vi "Main Page.vi"(8 "error in (no error)":errorcluster, 11 "Node Ptr":T11 format="%.0x") -> (0 "error out":errorcluster)   [LabVIEW 2018, in "Chassis TimeSync System Explorer.lvlib"]
uses:
  Chassis TimeSync System Explorer.lvlib
  <vilib>/NI Veristand/Custom Device API/Custom Device Item Ref.ctl
  Connection Selection.ctl
  Shared/Routes.ctl
  Shared/Route.ctl
  Pins Tab.ctl
  Shared/Mode.ctl
  Shared/External Pin.ctl
  Shared/Time Reference.ctl
  Time Ref Tab.ctl
  Shared/IRIG Type.ctl
  <vilib>/NI Veristand/Custom Device API/Custom Device Channel Type.ctl
  Shared/Constants.vi
  <vilib>/NI Veristand/Custom Device API/Get Item Property (Boolean).vi
  sub_EnableDisable Control.vi
  <vilib>/NI Veristand/Custom Device API/Get Item Property (String).vi
  <vilib>/NI Veristand/Custom Device API/Get Item Property (U16).vi
  <vilib>/NI Veristand/Custom Device API/Get Item Property (Double).vi
  <vilib>/NI Veristand/Custom Device API/Set Item Property (String).vi
  <vilib>/NI Veristand/Custom Device API/Set Item Property (Boolean).vi
  <vilib>/NI Veristand/Custom Device API/Set Item Property (Variant).vi
  <vilib>/NI Veristand/Custom Device API/Set Item Property (U16).vi
  <vilib>/NI Veristand/Custom Device API/Set Item Property (I32).vi
  <vilib>/NI Veristand/Custom Device API/Set Item Property (Double).vi
  <vilib>/NI Veristand/Custom Device API/Custom Device API.lvlib
  Shared/Chassis TimeSync Shared.lvlib
panel:
  in  "6683H Warning":string
  in  "SyncModule":string caption="Chassis Clock Generation Module"
  in  "SyncModule?":bool
  in  "Settings":T1(tab)
  out "Mode Desciption":string
  in  "Mode":T2
  in  "ConSelection":T3 caption="Selection"
  out "Pins tab":T4
  in  "PFI2":bool
  in  "PFI1":bool
  in  "PFI0":bool
  in  "PXI_Trig0":bool
  in  "Route In Pin":T5
  in  "Custom Routes":T6
  out "TimeRefTab":T8
  in  "Priority 2":i32 min=0 max=255
  in  "Priority 1":i32 min=0 max=255
  in  "IRIG type":T9=enum."IRIGB AM"
  in  "Start Time":timestamp
  in  "PPSSetTime":bool
  in  "Terminal":string
  in  "Time Reference":T10
  out "Mode Desciption 2":string="When using a time reference other than PXI Backplane Clock, it is recommended to additionally configure that time refernece in Measurment and Automation Explorer (MAX) before deployment. Doing so will prevent \"macro\" adjustments to system time while the NI VeriStand engine is running."
  in  "StartDelay":u16 caption="Generation Start Delay (s)"
  in  "PhaseOffset":dbl caption="Generation Phase Offset (°)" min=0.0 max=360.0
  in  "timekeeper":string caption="Time-Based Synchronization Module"
  in  "Header":cluster{"Section Name":string}={"Section Name"="Chassis TimeSync Settings"}
  in  "Description":string
  in  "Name":string
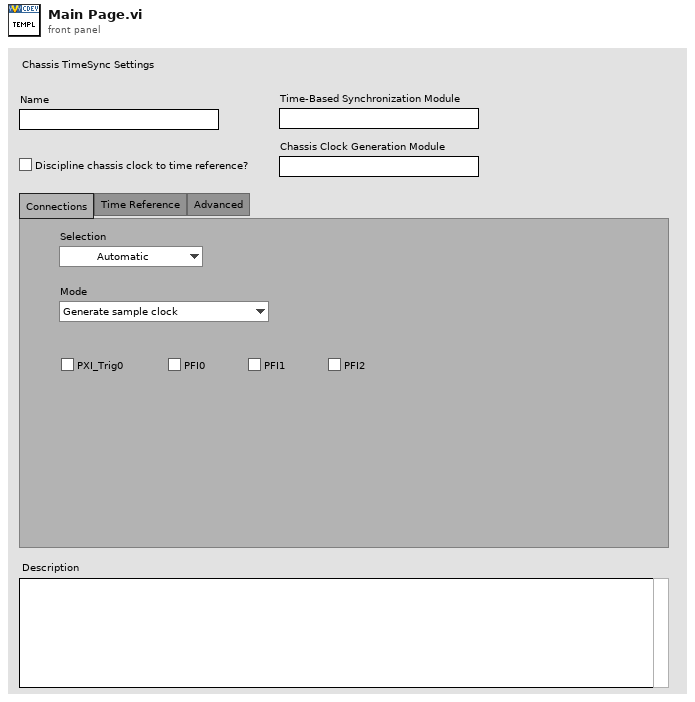
[diagram p1: front panel]
types:
  T1 = enum32{"Connections", "Time Reference", "Advanced"}
  T2 = typedef "Chassis TimeSync Shared.lvlib/Mode.ctl" = enum16{"Generate sample clock", "Route sample clock out of chassis", "Route sample clock into chassis", "Custom routes"}
  T3 = typedef "Chassis TimeSync System Explorer.lvlib/Connection Selection.ctl" = enum16{"Automatic", "Custom"}
  T4 = typedef "Chassis TimeSync System Explorer.lvlib/Pins Tab.ctl" = enum32{"Pins", "Ext. Pin", "Custom"}
  T5 = typedef "Chassis TimeSync Shared.lvlib/External Pin.ctl" = enum16{"PFI0", "PFI1", "PFI2"}
  T6 = typedef "Chassis TimeSync Shared.lvlib/Routes.ctl" = T7[]
  T7 = typedef "Chassis TimeSync Shared.lvlib/Route.ctl" = cluster{"Source":string, "Destination":string}
  T8 = typedef "Chassis TimeSync System Explorer.lvlib/Time Ref Tab.ctl" = enum32{"Empty", "1588", "IRIG", "PPS"}
  T9 = typedef "Chassis TimeSync Shared.lvlib/IRIG Type.ctl" = enum16{"IRIGB DC", "IRIGB AM"}
  T10 = typedef "Chassis TimeSync Shared.lvlib/Time Reference.ctl" = enum16{"GPS", "IRIG", "PPS", "1588 Ordinary Clock", "802.1AS", "PXI Chassis Clock", "Free Running (Internal)"}
  T11 = typedef "Custom Device API.lvlib/Custom Device Item Ref.ctl" = u64
  T12 = typedef "Chassis TimeSync Shared.lvlib/Connection Settings.ctl" = cluster{"Mode":T2, "pxitrig":bool, "pfi0":bool, "pfi1":bool, "pfi2":bool, "External Pin":T5, "Routes":T6}
  T13 = typedef "Custom Device API.lvlib/Custom Device Item Info.ctl" = cluster{"Name":string, "Is Channel":bool, "GUID":string, "Is Waveform":bool}
  T14 = typedef "Chassis TimeSync Shared.lvlib/Time Ref Settings.ctl" = cluster{"Time Reference":T10, "Priority 1":i32, "Priority 2":i32, "IRIG type":T9, "Terminal":string, "PPSSetTime":bool, "Start Time":timestamp}
  T15 = typedef "Custom Device API.lvlib/Custom Device Channel Type.ctl" = enum16{"Input", "Output"}
  T16 = typedef "Custom Device API.lvlib/Custom Device Commands.ctl" = enum16{"Default", "Item renamed", "Shutdown", "Dynamic button pressed"}
  T17 = typedef "Chassis TimeSync Shared.lvlib/Channel.ctl" = cluster{"Name":string, "Units":string, "Default":dbl, "Description":string}
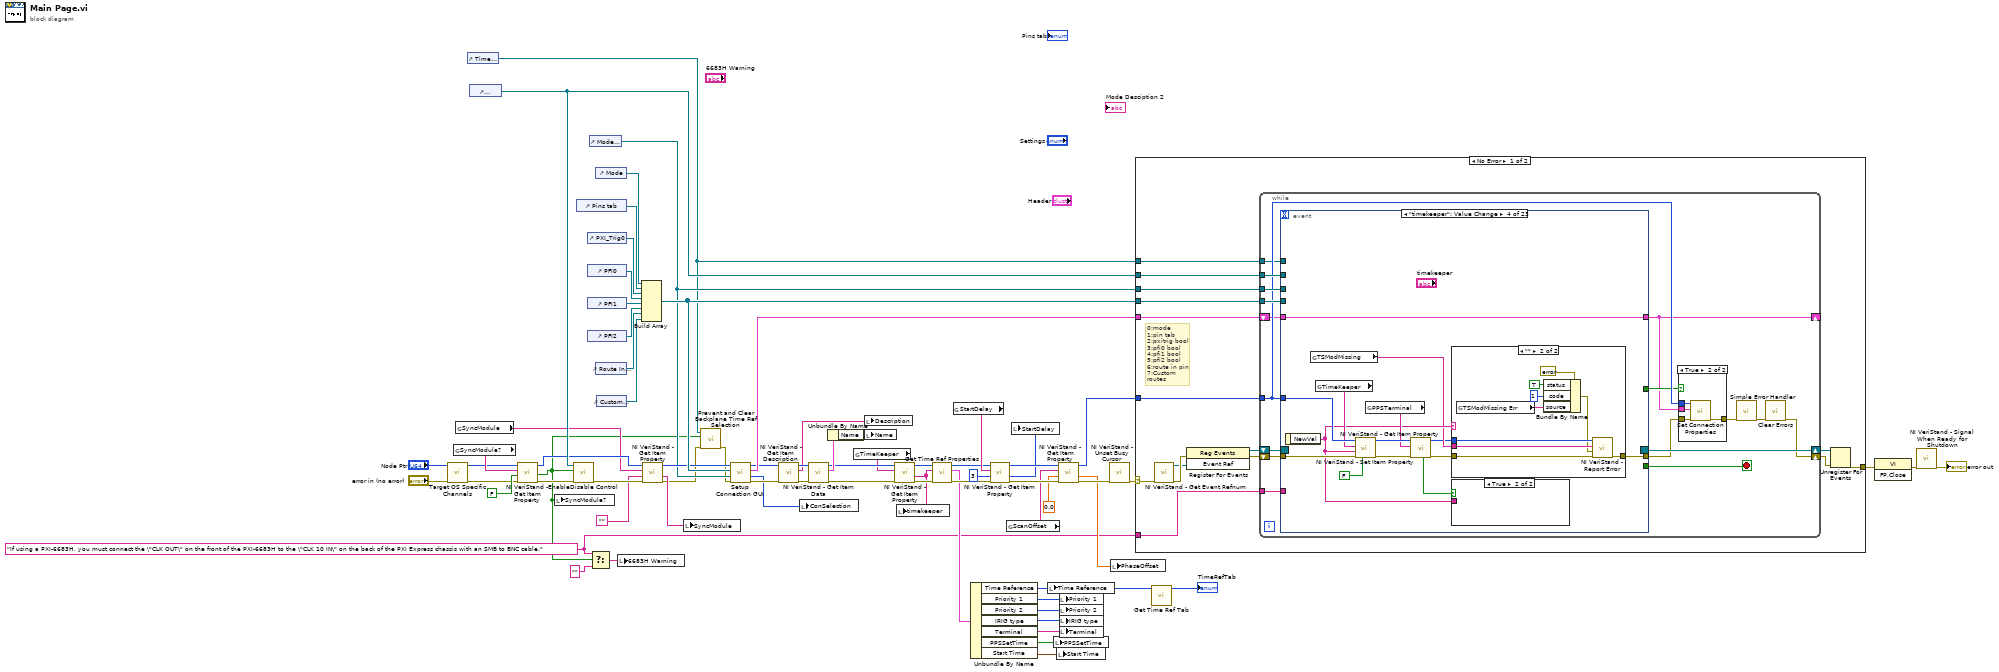
[diagram p0: block diagram]
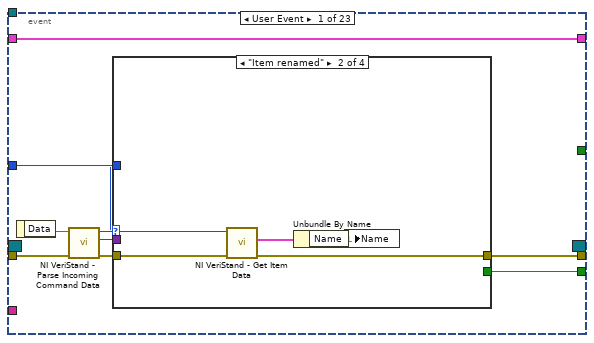
[diagram p3: hidden frame]
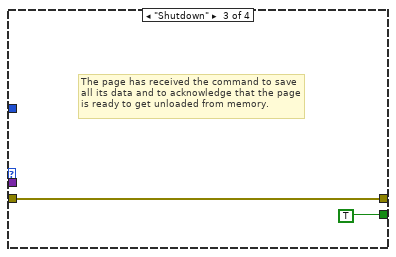
[diagram p5: hidden frame]
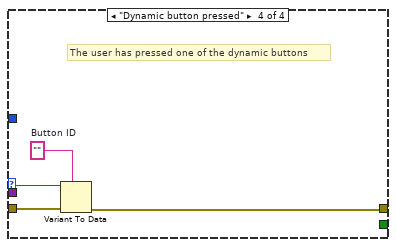
[diagram p6: hidden frame]
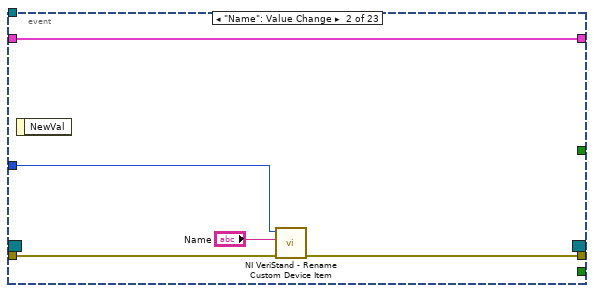
[diagram p7: hidden frame]
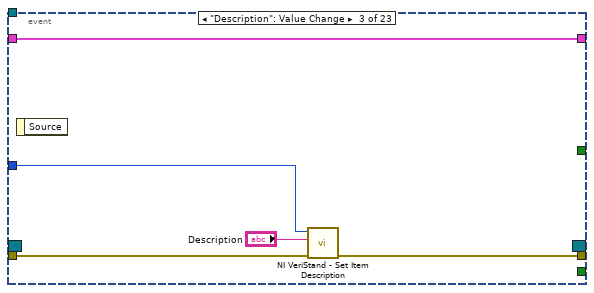
[diagram p8: hidden frame]
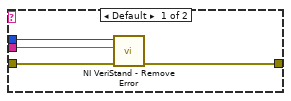
[diagram p9: hidden frame]
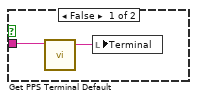
[diagram p10: hidden frame]
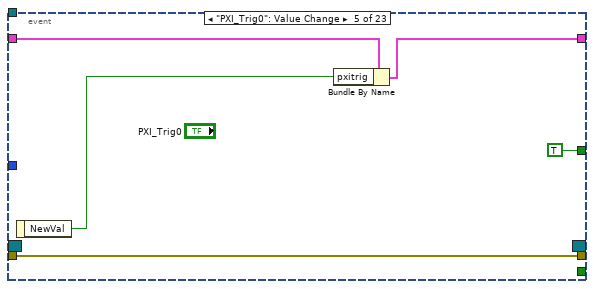
[diagram p11: hidden frame]
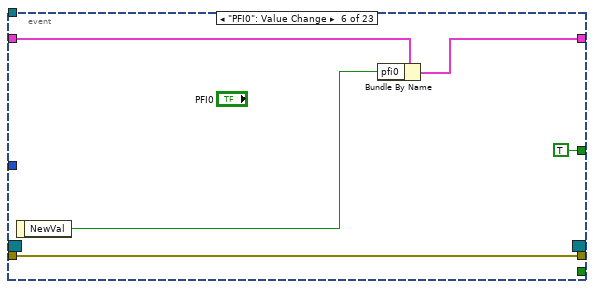
[diagram p12: hidden frame]
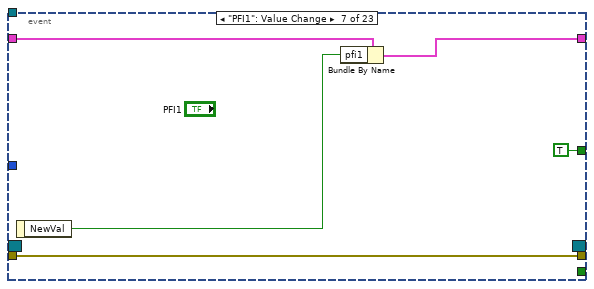
[diagram p13: hidden frame]
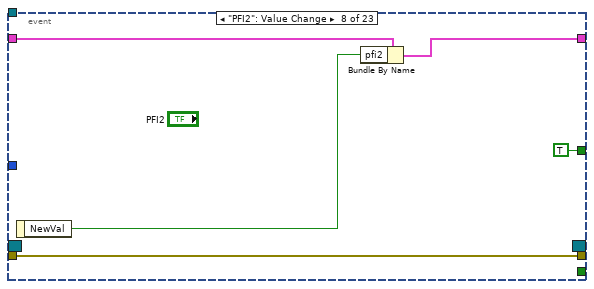
[diagram p14: hidden frame]
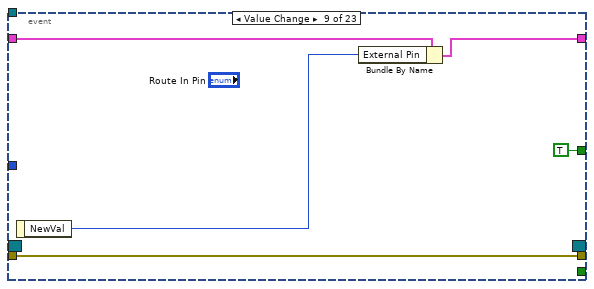
[diagram p15: hidden frame]
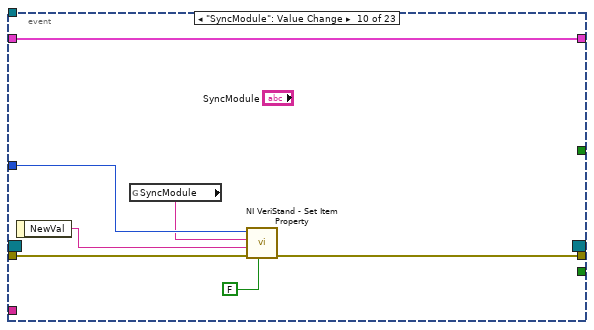
[diagram p16: hidden frame]
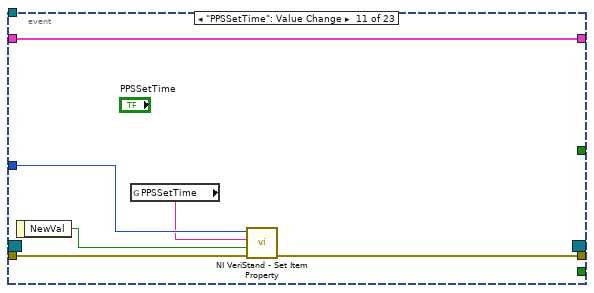
[diagram p17: hidden frame]
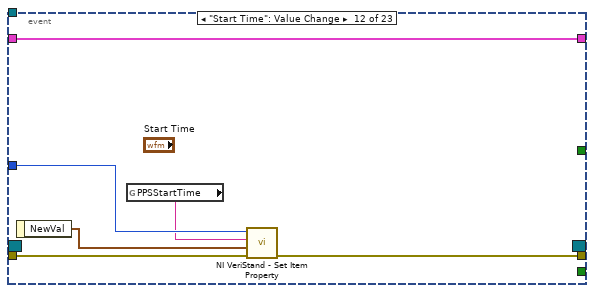
[diagram p18: hidden frame]
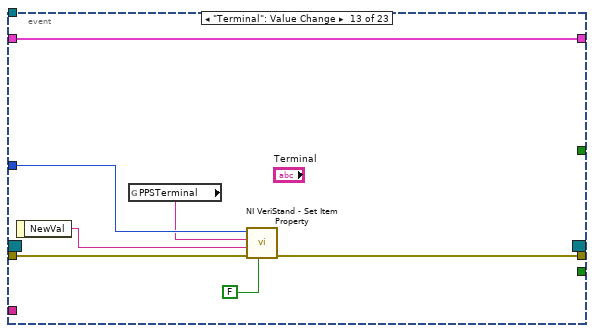
[diagram p19: hidden frame]
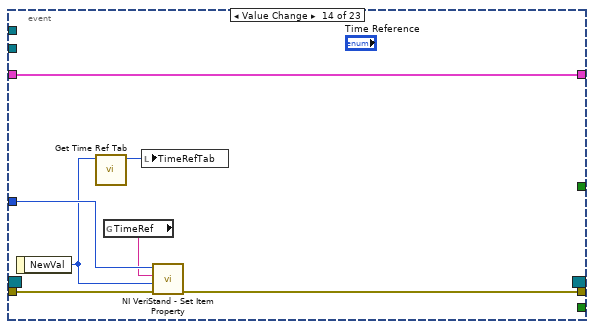
[diagram p20: hidden frame]
diagram:
  w5 = "If using a PXI-6683H, you must connect the \"CLK OUT\" on the front of the PXI-6683H to the \"CLK 10 IN\" on the back of the PXI Express chassis with an SMB to BNC cable." ("6683H Warning")
  n1 = call "Target OS Specific Channels.vi"("error in (no error)"="error in (no error)", "Device Item Ref in"="Node Ptr") -> ("error out"=w3:errorcluster, "Item Ref out"=w4:T11)  [unwired: 8 in]
  n2 = global read "Constants.vi" "SyncModule?"() -> (w37:string)
  n3 = global read "Constants.vi" "SyncModule"() -> (w32:string)
  n4 = control-ref of="Time Reference"() -> (w11:refnum<vi>)
  n5 = control-ref of="SyncModule"() -> (w34:refnum<vi>)
  n6 = call-poly <vilib>:"NI VeriStand - Get Item Property.vi"("error in (no error)"=w3, "Default Value"=FALSE, "Property Name"=w37, "Item Ref in"=w4) -> ("error out"=w38:errorcluster, "Value"=w8:bool, "Item Ref out"=w33:T11)  [unwired: 4 in, 1 out]
  n7 = local write "SyncModule?"(w8) -> ()
  n8 = call-poly "EnableDisable Control.vi"("error in (no error)"=w38, "Enable"=w8, "Control"=w34) -> ("error out"=w35:errorcluster)  [unwired: 8 in]
  n9 = control-ref of="Pins tab"() -> (w47:refnum<vi>)
  n10 = control-ref of="PXI_Trig0"() -> (w46:refnum<vi>)
  n11 = control-ref of="PFI0"() -> (w45:refnum<vi>)
  n12 = control-ref of="PFI1"() -> (w41:refnum<vi>)
  n13 = control-ref of="PFI2"() -> (w42:refnum<vi>)
  n14 = control-ref of="Mode Desciption"() -> (w12:refnum<vi>)
  n15 = Select(t=w5, s=w8, f="" ("6683H Warning")) -> (s? t:f=w6:string)
  n16 = control-ref of="Mode"() -> (w48:refnum<vi>)
  n17 = control-ref of="Route In Pin"() -> (w44:refnum<vi>)
  n18 = control-ref of="Custom Routes"() -> (w43:refnum<vi>)
  n19 = local write "6683H Warning"(w6) -> ()
  n20 = Build Array(w48, w47, w46, w45, w41, w42, w44, w43) -> (w39:refnum<vi>[])
  n21 = call-poly <vilib>:"NI VeriStand - Get Item Property.vi"("error in (no error)"=w35, "Default Value"="", "Property Name"=w32, "Item Ref in"=w33) -> ("error out"=w10:errorcluster, "Value"=w30:string, "Item Ref out"=w13:T11)  [unwired: 4 in, 1 out]
  n22 = local write "SyncModule"(w30) -> ()
  n23 = call "Prevent and Clear Backplane Time Ref Selection.vi"("error in (no error)"=w10, "Sync Mod?"=w8, "Time Reference Enum"=w11) -> ("error out"=w9:errorcluster)  [unwired: 8 in]
  n24 = call "Setup Connection GUI.vi"("error in (no error)"=w9, "Mode Description Control"=w12, "Connection Controls"=w39, "Item Ref in"=w13) -> ("error out"=w40:errorcluster, "ConSelection"=w16:T3, "Connection Settings"=w15:T12, "Item Ref out"=w14:T11)  [unwired: 4 in]
  n25 = call <vilib>:"NI VeriStand - Get Item Description.vi"("error in (no error)"=w40, "Item Ref in"=w14) -> ("error out"=w65:errorcluster, "Description"=w66:string, "Item Ref out"=w67:T11)  [unwired: 7 out]
  n26 = local write "ConSelection"(w16) -> ()
  n27 = call <vilib>:"NI VeriStand - Get Item Data.vi"("error in (no error)"=w65, "Item Ref in"=w67) -> ("error out"=w62:errorcluster, "Item Info"=w64:T13, "Item Ref out"=w61:T11)  [unwired: 7 out]
  n28 = Unbundle By Name(w64) -> ("Name"=w63:string)
  n29 = global read "Constants.vi" "TimeKeeper"() -> (w60:string)
  n30 = local write "Description"(w66) -> ()
  n31 = local write "Name"(w63) -> ()
  n32 = call-poly <vilib>:"NI VeriStand - Get Item Property.vi"("error in (no error)"=w62, "Property Name"=w60, "Item Ref in"=w61) -> ("error out"=w59:errorcluster, "Value"=w26:string, "Item Ref out"=w28:T11)  [unwired: 5 in, 1 out]
  n33 = local write "timekeeper"(w26) -> ()
  n34 = call "Get Time Ref Properties.vi"("error in (no error)"=w59, "TimeKeeper Module"=w26, "Device Item Ref in"=w28) -> ("error out"=w29:errorcluster, "Time Ref Settings"=w25:T14, "Item Ref out"=w27:T11)  [unwired: 6 in]
  n35 = global read "Constants.vi" "StartDelay"() -> (w54:string)
  n36 = Unbundle By Name(w25) -> ("Time Reference"=w18:T10, "Priority 1"=w24:i32, "Priority 2"=w23:i32, "IRIG type"=w22:T9, "Terminal"=w21:string, "PPSSetTime"=w20:bool, "Start Time"=w19:timestamp)
  n37 = call-poly <vilib>:"NI VeriStand - Get Item Property.vi"("error in (no error)"=w29, "Default Value"=u16 3 ("Start Offset Multiple"), "Property Name"=w54, "Item Ref in"=w27) -> ("error out"=w55:errorcluster, "Value"=w52:u16, "Item Ref out"=w58:T11)  [unwired: 4 in, 1 out]
  n38 = global read "Constants.vi" "ScanOffset"() -> (w51:string)
  n39 = local write "StartDelay"(w52) -> ()
  n40 = local write "Time Reference"(w18) -> ()
  n41 = local write "PPSSetTime"(w20) -> ()
  n42 = local write "Start Time"(w19) -> ()
  n43 = call-poly <vilib>:"NI VeriStand - Get Item Property.vi"("error in (no error)"=w55, "Default Value"=0.0 ("Scan Offset Scale (%)"), "Property Name"=w51, "Item Ref in"=w58) -> ("error out"=w56:errorcluster, "Value"=w49:dbl, "Item Ref out"=w57:T11)  [unwired: 4 in, 1 out]
  n44 = local write "Priority 1"(w24) -> ()
  n45 = local write "Priority 2"(w23) -> ()
  n46 = local write "IRIG type"(w22) -> ()
  n47 = local write "Terminal"(w21) -> ()
  n48 = call <vilib>:"NI VeriStand - Unset Busy Cursor.vi"("error in (no error)"=w56) -> ("error out"=w68:errorcluster)  [unwired: 10 out]
  n49 = local write "PhaseOffset"(w49) -> ()
  n50 = case shown="No Error" w68 {
    selector: w68 -> [w78 w332]
    tunnel: [w83 w330] -> w71
    tunnel: w57 -> [w79 _]
    tunnel: w39 -> [w77 _]
    tunnel: w12 -> [w76 _]
    tunnel: w34 -> [w75 _]
    tunnel: w15 -> [w74 _]
    tunnel: w11 -> [w73 _]
    tunnel: w5 -> [w72 _]
    frame No Error {
      # "0:mode\n1:pin tab\n2:pxitrig bool\n3:pfi0 bool\n4:pfi1 bool\n5:pfi2 bool\n6:route in pin\n7:Custom routes"
      n51 = call <vilib>:"NI VeriStand - Get Event Refnum.vi"("error in (no error)"=w78) -> ("error out"=w86:errorcluster, "Event Ref"=w82:refnum<user-event>)  [unwired: 9 out]
      n52 = register-events(error in=w86, w82) -> (reference out=w80:refnum<event-registration>, error out=w81:errorcluster)  [unwired: 1 in]
      n53 = while {
        tunnel: w79 -> [w92]
        shift-right: [w98] -> w84
        shift-left: w81 -> [w102]
        shift-right: [w103] -> w85
        shift-left: w80 -> [w101]
        tunnel: w77 -> [w97]
        tunnel: w76 -> [w96]
        tunnel: w75 -> [w95]
        shift-right: [w88] -> _
        shift-left: w74 -> [w91]
        tunnel: w73 -> [w89]
        tunnel: w72 -> [w87]
        stop <- w100 stop-if-true
        n54 = event shown="[3] \"timekeeper\": Value Change" {
          selector: w101 -> [_ _ _ _ _ _ _ _ _ _ _ _ _ _ _ _ _ _ _ _ _ _ _]
          dyn-events: [_ _ _ _ _ _ _ _ _ _ _ _ _ _ _ _ _ _ _ _ _ _ _] -> w103
          timeout: _ -> [_ _ _ _ _ _ _ _ _ _ _ _ _ _ _ _ _ _ _ _ _ _ _]
          tunnel: w102 -> [w117 w134 w138 w153 w173 w178 w183 w188 w193 w200 w206 w212 w219 w226 w232 w238 w244 w259 w277 w283 w289 w302 w325]
          tunnel: [w113 _ _ _ _ _ _ _ _ _ _ _ _ _ _ _ _ _ _ _ _ _ _] -> w100
          tunnel: [w112 w133 w137 w142 w173 w178 w183 w188 w193 w196 w202 w208 w215 w223 w228 w234 w240 w250 w277 w279 w285 w297 w322] -> w93
          tunnel: w92 -> [w111 w132 w139 w152 _ _ _ _ _ w199 w205 w211 w218 w225 w231 w237 w243 w251 _ w282 w288 w301 _]
          tunnel: w97 -> [_ _ _ _ _ _ _ _ _ _ _ _ _ _ _ _ _ _ _ _ _ w299 w323]
          tunnel: w96 -> [_ _ _ _ _ _ _ _ _ _ _ _ _ _ _ _ _ _ _ _ _ w298 _]
          tunnel: w95 -> [_ _ _ _ _ _ _ _ _ _ _ _ _ _ _ _ _ w256 _ _ _ _ _]
          tunnel: [w109 w130 w135 w150 w170 w176 w181 w186 w191 w195 w201 w207 w214 w222 w227 w233 w239 w255 w275 w278 w284 w290 w311] -> w88
          tunnel: w91 -> [w109 w130 w135 w150 w171 w177 w182 w187 w192 w195 w201 w207 w214 w222 w227 w233 w239 w255 w276 w278 w284 w292 w312]
          tunnel: [_ _ _ _ TRUE TRUE TRUE TRUE TRUE _ _ _ _ _ _ _ _ _ TRUE _ _ _ TRUE] -> w90
          tunnel: w89 -> [_ _ _ _ _ _ _ _ _ _ _ _ _ _ _ _ _ w254 _ _ _ _ _]
          tunnel: w87 -> [_ _ _ _ _ _ _ _ _ _ _ _ _ _ _ _ _ w247 _ _ _ _ _]
          event User Event {
            n55 = event-data() -> ("Data"=w116:string)  [unwired: 1 out]
            n56 = call <vilib>:"NI VeriStand - Parse Incoming Command Data.vi"("error in (no error)"=w117, "Incoming data"=w116) -> ("error out"=w115:errorcluster, "Outgoing data"=w110:variant, "Action"=w114:T16)  [unwired: 7 out]
            n57 = case shown="\"Item renamed\"" w114 {
              tunnel: w115 -> [w118 w123 w124 w129]
              tunnel: [_ _ TRUE _] -> w113
              tunnel: [w118 w120 w124 w126] -> w112
              tunnel: w111 -> [_ w122 _ _]
              tunnel: w110 -> [_ _ _ w128]
              frame "Default", Default {
              }
              frame "Item renamed" {
                n58 = call <vilib>:"NI VeriStand - Get Item Data.vi"("error in (no error)"=w123, "Item Ref in"=w122) -> ("error out"=w120:errorcluster, "Item Info"=w121:T13)  [unwired: 8 out]
                n59 = Unbundle By Name(w121) -> ("Name"=w119:string)
                n60 = local write "Name"(w119) -> ()
              }
              frame "Shutdown" {
                # "The page has received the command to save all its data and to acknowledge that the page is ready to get unloaded from memory."
              }
              frame "Dynamic button pressed" {
                w127 = ""  # Button ID
                # "The user has pressed one of the dynamic buttons"
                n61 = Variant To Data(error in=w129, type=w127, Variant=w128) -> (error out=w126:errorcluster)  [unwired: 1 out]
              }
            }
          }
          event "Name": Value Change {
            n62 = event-data() -> ()  [unwired: 2 out]
            n63 = call <vilib>:"NI VeriStand - Rename Custom Device Item.vi"("error in (no error)"=w134, "New Name"="Name", "Item Ref in"=w132) -> ("error out"=w133:errorcluster)  [unwired: 1 in, 7 out]
          }
          event "Description": Value Change {
            n64 = event-data() -> ()  [unwired: 2 out]
            n65 = call <vilib>:"NI VeriStand - Set Item Description.vi"("error in (no error)"=w138, "Description"="Description", "Item Ref in"=w139) -> ("error out"=w137:errorcluster)  [unwired: 8 out]
          }
          event "timekeeper": Value Change {
            n66 = event-data() -> ("NewVal"=w143:string)  [unwired: 1 out]
            n67 = global read "Constants.vi" "TSModMissing"() -> (w141:string)
            n68 = global read "Constants.vi" "TimeKeeper"() -> (w151:string)
            n69 = call-poly <vilib>:"NI VeriStand - Set Item Property.vi"("Binary String (T)"=FALSE, "error in (no error)"=w153, "Value"=w143, "Property Name"=w151, "Item Ref in"=w152) -> ("error out"=w148:errorcluster, "Item Ref out"=w147:T11)  [unwired: 4 in, 1 out]
            n70 = global read "Constants.vi" "PPSTerminal"() -> (w146:string)
            n71 = call-poly <vilib>:"NI VeriStand - Get Item Property.vi"("error in (no error)"=w148, "Property Name"=w146, "Item Ref in"=w147) -> ("error out"=w144:errorcluster, "Item Ref out"=w140:T11, "Found?"=w145:bool)  [unwired: 5 in, 1 out]
            n72 = case shown="\"\"" w143 {
              tunnel: w144 -> [w157 w166]
              tunnel: [w154 w165] -> w142
              tunnel: w141 -> [w156 w164]
              tunnel: w140 -> [w155 w163]
              frame Default {
                n73 = call <vilib>:"NI VeriStand - Remove Error.vi"("error in (no error)"=w157, "Error ID"=w156, "Node Ref in"=w155) -> ("error out"=w154:errorcluster)  [unwired: 7 in, 1 out]
              }
              frame "" {
                n74 = global read "Constants.vi" "TSModMissing Err"() -> (w159:string)
                n75 = Bundle By Name(cluster=errorcluster {"status"=FALSE, "code"=0, "source"=""} ("error constant"), "status"=TRUE, "code"=1, "source"=w159) -> (w158:errorcluster)
                n76 = call <vilib>:"NI VeriStand - Report Error.vi"("error in (no error)"=w166, "New Error"=w158, "Error ID"=w164, "Node Ref in"=w163) -> ("error out"=w165:errorcluster)  [unwired: 6 in, 1 out]
              }
            }
            n77 = case shown="True" w145 {
              tunnel: w143 -> [w168 _]
              frame False {
                n78 = call "Get PPS Terminal Default.vi"("TimeKeeper Module"=w168) -> ("PPSTerminal Default"=w167:string)  [unwired: 10 in]
                n79 = local write "Terminal"(w167) -> ()
              }
              frame True {
              }
            }
          }
          event "PXI_Trig0": Value Change {
            n80 = event-data() -> ("NewVal"=w172:bool)  [unwired: 1 out]
            n81 = Bundle By Name(cluster=w171, "pxitrig"=w172) -> (w170:T12)
          }
          event "PFI0": Value Change {
            n82 = event-data() -> ("NewVal"=w175:bool)  [unwired: 1 out]
            n83 = Bundle By Name(cluster=w177, "pfi0"=w175) -> (w176:T12)
          }
          event "PFI1": Value Change {
            n84 = event-data() -> ("NewVal"=w180:bool)  [unwired: 1 out]
            n85 = Bundle By Name(cluster=w182, "pfi1"=w180) -> (w181:T12)
          }
          event "PFI2": Value Change {
            n86 = event-data() -> ("NewVal"=w185:bool)  [unwired: 1 out]
            n87 = Bundle By Name(cluster=w187, "pfi2"=w185) -> (w186:T12)
          }
          event Value Change {
            n88 = event-data() -> ("NewVal"=w190:T5)  [unwired: 1 out]
            n89 = Bundle By Name(cluster=w192, "External Pin"=w190) -> (w191:T12)
          }
          event "SyncModule": Value Change {
            n90 = event-data() -> ("NewVal"=w197:string)  [unwired: 1 out]
            n91 = global read "Constants.vi" "SyncModule"() -> (w198:string)
            n92 = call-poly <vilib>:"NI VeriStand - Set Item Property.vi"("Binary String (T)"=FALSE, "error in (no error)"=w200, "Value"=w197, "Property Name"=w198, "Item Ref in"=w199) -> ("error out"=w196:errorcluster)  [unwired: 4 in, 2 out]
          }
          event "PPSSetTime": Value Change {
            n93 = event-data() -> ("NewVal"=w203:bool)  [unwired: 1 out]
            n94 = global read "Constants.vi" "PPSSetTime"() -> (w204:string)
            n95 = call-poly <vilib>:"NI VeriStand - Set Item Property.vi"("error in (no error)"=w206, "Value"=w203, "Property Name"=w204, "Item Ref in"=w205) -> ("error out"=w202:errorcluster)  [unwired: 5 in, 2 out]
          }
          event "Start Time": Value Change {
            n96 = event-data() -> ("NewVal"=w209:timestamp)  [unwired: 1 out]
            n97 = global read "Constants.vi" "PPSStartTime"() -> (w210:string)
            n98 = call-poly <vilib>:"NI VeriStand - Set Item Property.vi"("error in (no error)"=w212, "Value"=w209, "Property Name"=w210, "Item Ref in"=w211) -> ("error out"=w208:errorcluster)  [unwired: 5 in, 2 out]
          }
          event "Terminal": Value Change {
            n99 = event-data() -> ("NewVal"=w216:string)  [unwired: 1 out]
            n100 = global read "Constants.vi" "PPSTerminal"() -> (w217:string)
            n101 = call-poly <vilib>:"NI VeriStand - Set Item Property.vi"("Binary String (T)"=FALSE, "error in (no error)"=w219, "Value"=w216, "Property Name"=w217, "Item Ref in"=w218) -> ("error out"=w215:errorcluster)  [unwired: 4 in, 2 out]
          }
          event Value Change {
            n102 = event-data() -> ("NewVal"=w221:T10)  [unwired: 1 out]
            n103 = call "Get Time Ref Tab.vi"("Time Ref"=w221) -> ("TimeRefTab"=w220:T8)  [unwired: 10 in]
            n104 = global read "Constants.vi" "TimeRef"() -> (w224:string)
            n105 = local write "TimeRefTab"(w220) -> ()
            n106 = call-poly <vilib>:"NI VeriStand - Set Item Property.vi"("error in (no error)"=w226, "Value"=w221, "Property Name"=w224, "Item Ref in"=w225) -> ("error out"=w223:errorcluster)  [unwired: 5 in, 2 out]
          }
          event Value Change {
            n107 = event-data() -> ("NewVal"=w229:T9)  [unwired: 1 out]
            n108 = global read "Constants.vi" "IRIGType"() -> (w230:string)
            n109 = call-poly <vilib>:"NI VeriStand - Set Item Property.vi"("error in (no error)"=w232, "Value"=w229, "Property Name"=w230, "Item Ref in"=w231) -> ("error out"=w228:errorcluster)  [unwired: 5 in, 2 out]
          }
          event "Priority 1": Value Change {
            n110 = event-data() -> ("NewVal"=w235:i32)  [unwired: 1 out]
            n111 = global read "Constants.vi" "Priority1"() -> (w236:string)
            n112 = call-poly <vilib>:"NI VeriStand - Set Item Property.vi"("error in (no error)"=w238, "Value"=w235, "Property Name"=w236, "Item Ref in"=w237) -> ("error out"=w234:errorcluster)  [unwired: 5 in, 2 out]
          }
          event "Priority 2": Value Change {
            n113 = event-data() -> ("NewVal"=w241:i32)  [unwired: 1 out]
            n114 = global read "Constants.vi" "Priority2"() -> (w242:string)
            n115 = call-poly <vilib>:"NI VeriStand - Set Item Property.vi"("error in (no error)"=w244, "Value"=w241, "Property Name"=w242, "Item Ref in"=w243) -> ("error out"=w240:errorcluster)  [unwired: 5 in, 2 out]
          }
          event "SyncModule?": Value Change {
            n116 = event-data() -> ("NewVal"=w248:bool)  [unwired: 1 out]
            n117 = global read "Constants.vi" "SyncModule?"() -> (w258:string)
            n118 = call-poly <vilib>:"NI VeriStand - Set Item Property.vi"("error in (no error)"=w259, "Value"=w248, "Property Name"=w258, "Item Ref in"=w251) -> ("error out"=w257:errorcluster)  [unwired: 5 in, 2 out]
            n119 = Select(t=w247, s=w248, f="") -> (s? t:f=w245:string)
            n120 = call-poly "EnableDisable Control.vi"("error in (no error)"=w257, "Enable"=w248, "Control"=w256) -> ("error out"=w253:errorcluster)  [unwired: 8 in]
            n121 = local write "6683H Warning"(w245) -> ()
            n122 = call "Prevent and Clear Backplane Time Ref Selection.vi"("error in (no error)"=w253, "Sync Mod?"=w248, "Time Reference Enum"=w254) -> ("error out"=w252:errorcluster)  [unwired: 8 in]
            n123 = global read "Constants.vi" "Chassis Clock Section"() -> (w249:string)
            n124 = case shown="False" w248 {
              tunnel: w252 -> [w266 w272]
              tunnel: w251 -> [w265 w271]
              tunnel: [w260 w268] -> w250
              tunnel: w249 -> [w264 w267]
              frame False {
                n125 = call <vilib>:"NI VeriStand - Get Item Reference by Name.vi"("error in (no error)"=w266, "Item Name"=w264, "Parent Ref in"=w265) -> ("error out"=w263:errorcluster, "Item Ref"=w262:T11)  [unwired: 5 in, 2 out]
                n126 = call <vilib>:"NI VeriStand - Remove Custom Device Item.vi"("error in (no error)"=w263, "Force Delete (F)"=TRUE, "Item Ref in"=w262) -> ("error out"=w260:errorcluster)  [unwired: 7 in, 1 out]
              }
              frame True {
                n127 = global read "Constants.vi" "ChassisClk Chans"() -> (w269:T17[])
                n128 = call "Create Chans.vi"("New Section Name (none)"=w267, "Type"=Custom_Device_Channel_Type."Output", "error in (no error)"=w272, "Channels"=w269, "Section Ptr"=w271) -> ("error out"=w268:errorcluster)  [unwired: 5 in, 1 out]
              }
            }
          }
          event Value Change {
            n129 = event-data() -> ("NewVal"=w274:T6)  [unwired: 1 out]
            n130 = Bundle By Name(cluster=w276, "Routes"=w274) -> (w275:T12)
          }
          event "PhaseOffset": Value Change {
            n131 = event-data() -> ("NewVal"=w280:dbl)  [unwired: 1 out]
            n132 = global read "Constants.vi" "ScanOffset"() -> (w281:string)
            n133 = call-poly <vilib>:"NI VeriStand - Set Item Property.vi"("error in (no error)"=w283, "Value"=w280, "Property Name"=w281, "Item Ref in"=w282) -> ("error out"=w279:errorcluster)  [unwired: 5 in, 2 out]
          }
          event "StartDelay": Value Change {
            n134 = event-data() -> ("NewVal"=w286:u16)  [unwired: 1 out]
            n135 = global read "Constants.vi" "StartDelay"() -> (w287:string)
            n136 = call-poly <vilib>:"NI VeriStand - Set Item Property.vi"("error in (no error)"=w289, "Value"=w286, "Property Name"=w287, "Item Ref in"=w288) -> ("error out"=w285:errorcluster)  [unwired: 5 in, 2 out]
          }
          event Value Change {
            n137 = event-data() -> ("NewVal"=w295:T3)  [unwired: 1 out]
            n138 = global read "Constants.vi" "ConSelection"() -> (w300:string)
            n139 = call-poly <vilib>:"NI VeriStand - Set Item Property.vi"("error in (no error)"=w302, "Value"=w295, "Property Name"=w300, "Item Ref in"=w301) -> ("error out"=w296:errorcluster, "Item Ref out"=w293:T11)  [unwired: 5 in, 1 out]
            n140 = case shown="\"Custom\"" w295 {
              tunnel: w296 -> [w304 w309]
              tunnel: [w304 w308] -> w294
              tunnel: w293 -> [w303 w307]
              tunnel: w292 -> [_ w306]
              tunnel: [w303 w305] -> w291
              frame "Automatic" {
              }
              frame "Custom" {
                n141 = call "Set Connection Properties.vi"("error in (no error)"=w309, "AutoSelect"=w306, "Device Item Ref in"=w307) -> ("error out"=w308:errorcluster, "Item Ref out"=w305:T11)  [unwired: 7 in]
              }
            }
            n142 = call "Setup Connection GUI.vi"("error in (no error)"=w294, "Mode Description Control"=w298, "Connection Controls"=w299, "Item Ref in"=w291) -> ("error out"=w297:errorcluster, "Connection Settings"=w290:T12)  [unwired: 4 in, 2 out]
          }
          event Value Change {
            n143 = event-data() -> ("NewVal"=w315:T2)  [unwired: 1 out]
            n144 = Equal?(x=w315, y=Mode."Route sample clock out of chassis" ("x")) -> (x = y?=w313:bool)
            n145 = Equal?(x=w315, y=Mode."Generate sample clock" ("x")) -> (x = y?=w317:bool)
            n146 = Index Array(array=w323, index=2) -> (element=w319:refnum<vi>)
            n147 = call "Get Connection Description Text and Pins Tab.vi"("Mode"=w315) -> ("Pins tab"=w321:T4, "Description"=→"Mode Desciption":string)  [unwired: 9 in]
            n148 = local write "Pins tab"(w321) -> ()
            n149 = call-poly "EnableDisable Control.vi"("error in (no error)"=w325, "Enable"=w317, "Control"=w319) -> ("error out"=w322:errorcluster)  [unwired: 8 in]
            n150 = Bundle By Name(cluster=w312, "Mode"=w315) -> (w310:T12)
            n151 = case shown="True" w313 {
              tunnel: w310 -> [w326 w329]
              tunnel: [w326 w328] -> w311
              frame False {
              }
              frame True {
                n152 = Bundle By Name(cluster=w329, "pxitrig"=FALSE) -> (w328:T12)
              }
            }
          }
        }
        n153 = case shown="True" w90 {
          tunnel: [w104 w108] -> w94
          tunnel: w93 -> [w104 w107]
          tunnel: w92 -> [_ w106]
          tunnel: w88 -> [_ w105]
          frame False {
          }
          frame True {
            n154 = call "Set Connection Properties.vi"("error in (no error)"=w107, "AutoSelect"=w105, "Device Item Ref in"=w106) -> ("error out"=w108:errorcluster)  [unwired: 7 in, 1 out]
          }
        }
        n155 = call <vilib>:"Simple Error Handler.vi"("error in (no error)"=w94) -> ("error out"=w99:errorcluster)  [unwired: 1 in, 7 out]
        n156 = call <vilib>:"Clear Errors.vi"("error in (no error)"=w99) -> ("error out"=w98:errorcluster)  [unwired: 1 in, 5 out]
      }
      n157 = Unregister For Events(event registration refnum=w85, error in=w84) -> (error out=w83:errorcluster)
    }
    frame Error {
      n158 = call <vilib>:"Simple Error Handler.vi"("error in (no error)"=w332) -> ("error out"=w331:errorcluster)  [unwired: 1 in, 7 out]
      n159 = call <vilib>:"Clear Errors.vi"("error in (no error)"=w331) -> ("error out"=w330:errorcluster)  [unwired: 1 in, 5 out]
    }
  }
  n160 = call "Get Time Ref Tab.vi"("Time Ref"=w18) -> ("TimeRefTab"=→"TimeRefTab":T8)  [unwired: 10 in]
  n161 = invoke class="VI" method="FP.Close"(error in=w71) -> (error out=w70:errorcluster)  [unwired: 2 in, 2 out]
  n162 = call <vilib>:"NI VeriStand - Signal When Ready for Shutdown.vi"("error in (no error)"=w70) -> ("error out"=→"error out":errorcluster)  [unwired: 10 out]
